vi "总磷氨氮插入数据.vi"(0 "table":string, 1 "关键参数":T1, 5 "data":T3={"时间标识"=timestamp(0 s since 1904-01-01), "测量模式"=enum."水样测试", "数据标记表"="N", "监测值"=0.0, "单位"=0, "数据标识"="", "因子编码"=0, "标样参考值"=0.0, "F0"=0.0, "F1"=0.0, "F2"=0.0, "F3"=0.0, "F4"=0.0, "F5"=0.0, "F6"=0.0, "F7"=0.0, "X"=0.0, "温度"=0.0, "湿度"=0.0, "量程标识"="", "SN"="", "跨度值"=0.0} {"单位" items=["μg/L", "mg/L", "ppm", "mg/m3", "cm", "ppb", "μg/m3", "%", "nmol/mol", "μmol/mol", "MPN/L", "MPN/100ml", "ng/m3", "NTU", "无量纲", "ms/cm", "μs/cm"]}, 11 "error in (no error)":errorcluster) -> (15 "error out":errorcluster)   [LabVIEW 2016, in "斯坦道氨氮.lvlib"]
uses:
  <vilib>/Utility/sysdir.llb/System Directory Type.ctl
  <vilib>/Utility/error.llb/DialogType.ctl
  <vilib>/addons/database/Auxilliary.llb/DB Tools Column Info.ctl
  <vilib>/addons/database/Auxilliary.llb/DB Tools DataTypes.ctl
  <vilib>/addons/database/Connection.llb/DB Tools Open Connec (String).vi
  <vilib>/addons/database/Connection.llb/Conn Execute.vi
  <vilib>/addons/database/Recordset.llb/Rec Fetch Recordset Data (R).vi
  <vilib>/addons/database/Recordset.llb/Rec Destroy - Connection.vi
  <vilib>/addons/database/NI_Database_API.lvlib
  <vilib>/Utility/VariantDataType/VariantType.lvlib
panel:
  out "data输出":T2
  out "为空？":bool
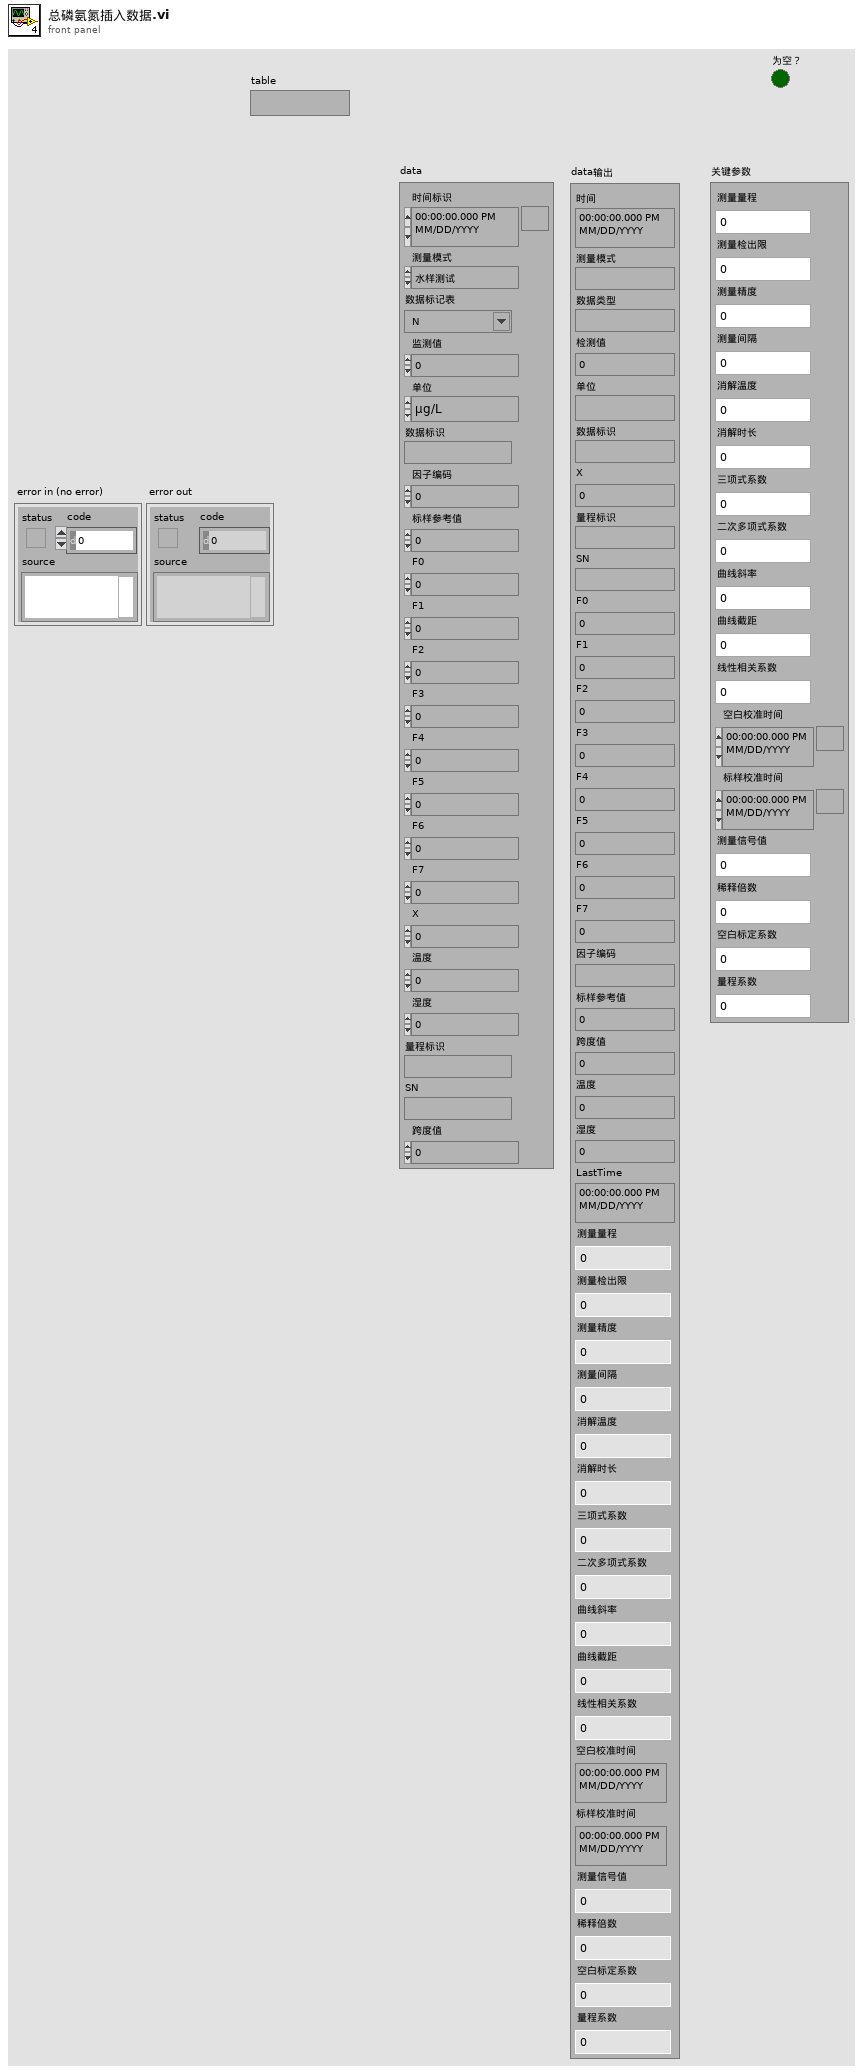
[diagram p1: front panel]
types:
  T1 = typedef "斯坦道氨氮.lvlib/关键参数.ctl" = cluster{"测量量程":sgl, "测量检出限":sgl, "测量精度":sgl, "测量间隔":sgl, "消解温度":sgl, "消解时长":sgl, "三项式系数":sgl, "二次多项式系数":sgl, "曲线斜率":sgl, "曲线截距":sgl, "线性相关系数":sgl, "空白校准时间":timestamp, "标样校准时间":timestamp, "测量信号值":sgl, "稀释倍数":sgl, "空白标定系数":sgl, "量程系数":sgl}
  T2 = cluster{"时间":timestamp, "测量模式":string, "数据类型":string, "检测值":sgl, "单位":string, "数据标识":string, "X":sgl, "量程标识":string, "SN":string, "F0":sgl, "F1":sgl, "F2":sgl, "F3":sgl, "F4":sgl, "F5":sgl, "F6":sgl, "F7":sgl, "因子编码":string, "标样参考值":sgl, "跨度值":sgl, "温度":sgl, "湿度":sgl, "LastTime":timestamp, "测量量程":sgl, "测量检出限":sgl, "测量精度":sgl, "测量间隔":sgl, "消解温度":sgl, "消解时长":sgl, "三项式系数":sgl, "二次多项式系数":sgl, "曲线斜率":sgl, "曲线截距":sgl, "线性相关系数":sgl, "空白校准时间":timestamp, "标样校准时间":timestamp, "测量信号值":sgl, "稀释倍数":sgl, "空白标定系数":sgl, "量程系数":sgl}
  T3 = cluster{"时间标识":timestamp, "测量模式":enum16{"维护数据", "水样测试", "标样核查", "零点核查", "跨度核查", "空白测试", "平行样测试", "加标回收", "空白校准", "标样校准", "初始化（清洗）", "快捷测试"}, "数据标记表":string, "监测值":sgl, "单位":u16, "数据标识":string, "因子编码":u32, "标样参考值":sgl, "F0":sgl, "F1":sgl, "F2":sgl, "F3":sgl, "F4":sgl, "F5":sgl, "F6":sgl, "F7":sgl, "X":sgl, "温度":sgl, "湿度":sgl, "量程标识":string, "SN":string, "跨度值":sgl}
  T4 = typedef "DialogType.ctl" = u16
  T5 = typedef "System Directory Type.ctl" = i32
  T6 = typedef "NI_Database_API.lvlib/Conn ObjectReference.ctl" = refnum<k1>
  T7 = typedef "NI_Database_API.lvlib/Rec ObjectReference.ctl" = refnum<k1>
  T8 = cluster{"测量量程":dbl, "测量精度":dbl, "测量间隔":dbl, "消解温度":dbl, "消解时长":dbl, "空白校准时间":timestamp, "曲线截距":dbl, "曲线斜率":dbl, "测量检出限":dbl, "测量信号值":dbl, "线性相关系数":dbl, "二次多项式系数":dbl, "标样校准时间":timestamp, "稀释倍数":dbl, "三项式系数":dbl, "空白标定系数":dbl, "量程系数":dbl, "F0/ORPA":dbl, "F1/ORPB":dbl, "F2/ORPK":dbl, "F3":dbl, "F4":dbl, "F5":dbl, "F6":dbl, "F7":dbl, "X0/滴定数":dbl, "量程":dbl}
  T9 = typedef "NI_Database_API.lvlib/DB Tools Column Info.ctl" = cluster{"column name":string, "data type":T10, "size":i32, "allow null?":bool}
  T10 = typedef "NI_Database_API.lvlib/DB Tools DataTypes.ctl" = enum16{"String", "Long (I32)", "Single (SGL)", "Double (DBL)", "Date/Time", "Binary"}
  T11 = typedef "VariantType.lvlib/Type.ctl" = enum8{"Invalid Type", "Void", "I8", "I16", "I32", "I64", "U8", "U16", "U32", "U64", "Single Float", "Double Float", "Extended Float", "Single Complex", "Double Complex", "Extended Complex", "Enum U8", "Enum U16", "Enum U32", "Enum U64", "Single Float With Unit", "Double Float With Unit", "Extended Float With Unit", "Single Complex with Unit", "Double Complex with Unit", "Extended Complex with Unit", "Boolean", "String", "Path", "Picture", "Tag", "Array", "Cluster", "Variant", "LV Variant", "Waveform", "Timestamp", "Digital Waveform", "Digital Data", "ExpressData", "Refnum", "External Data", "VI", "Poly VI", "LabVIEW Class Instance", "Fixed Point"}
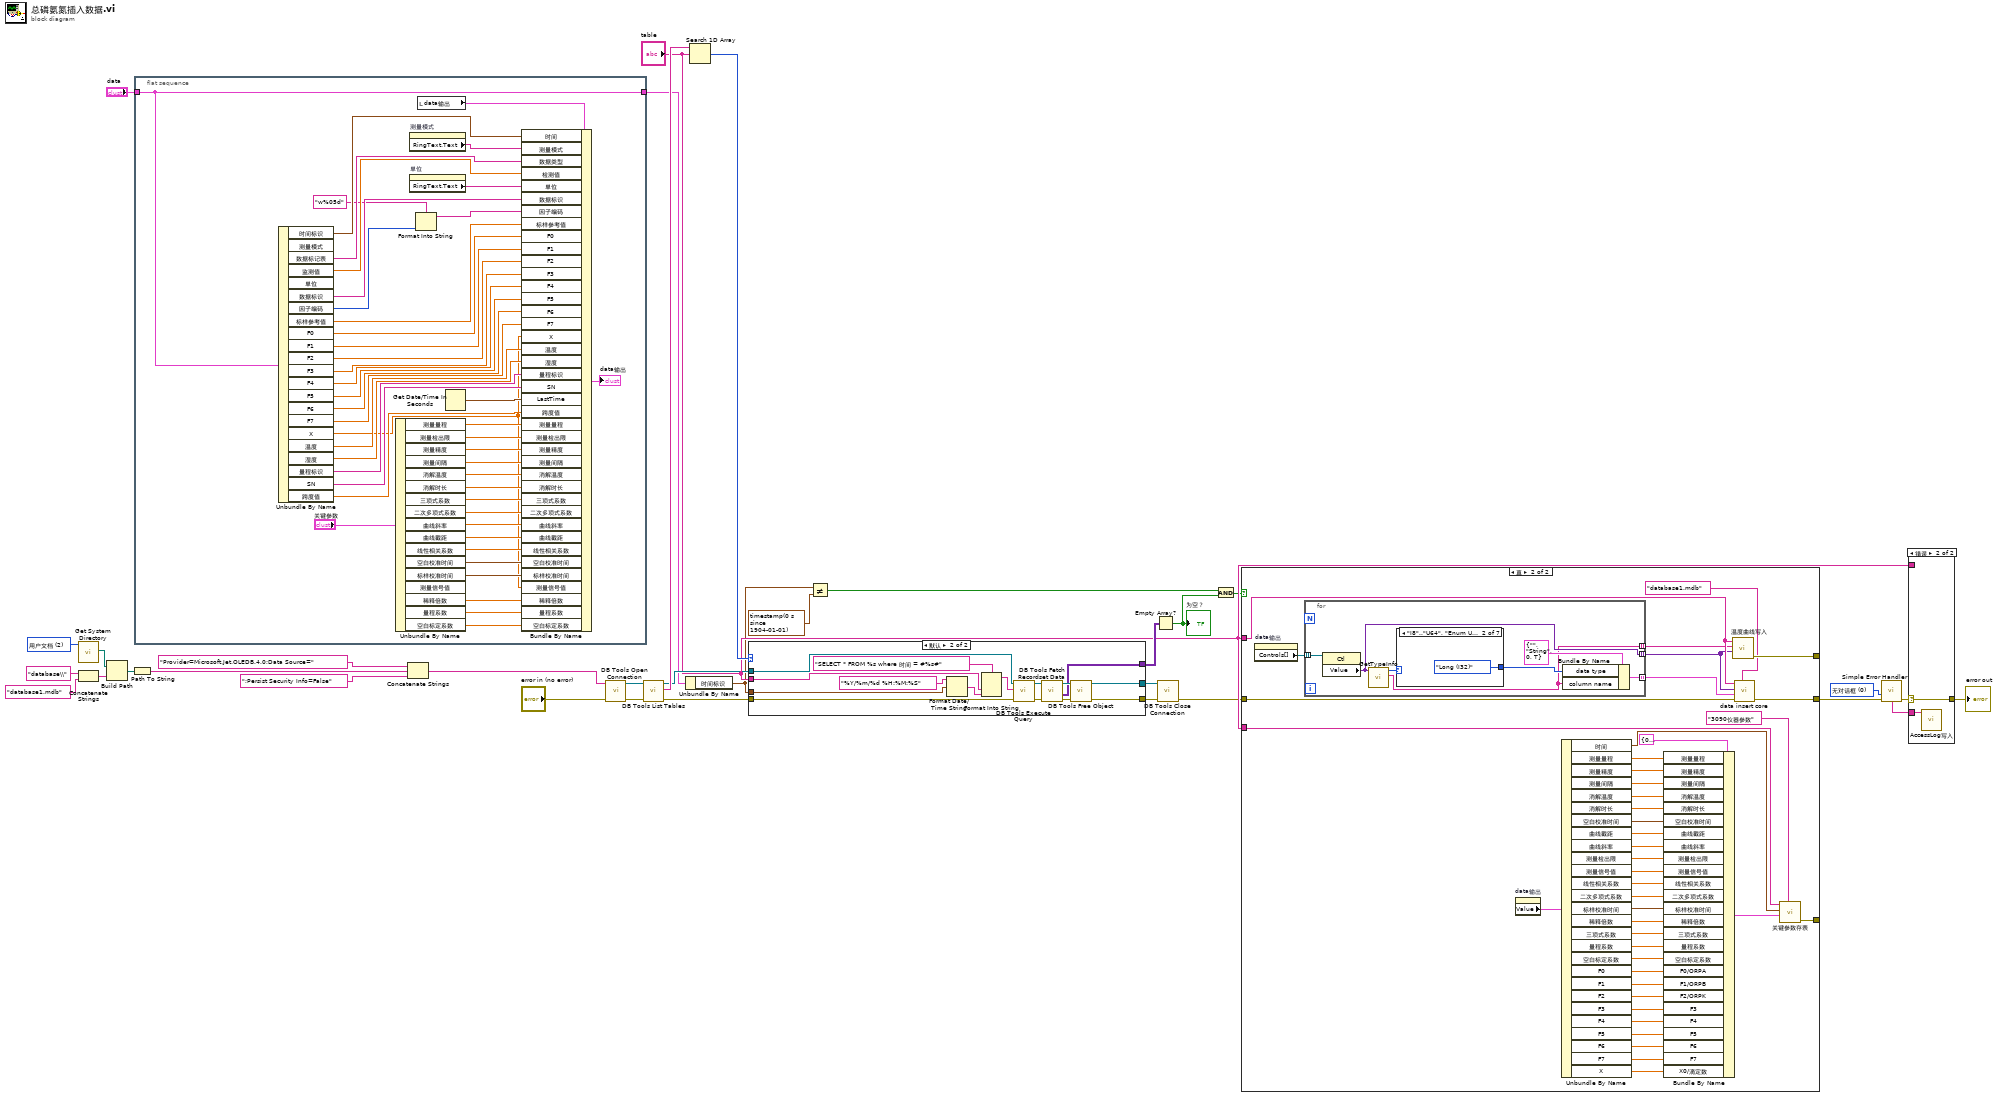
[diagram p0: block diagram]
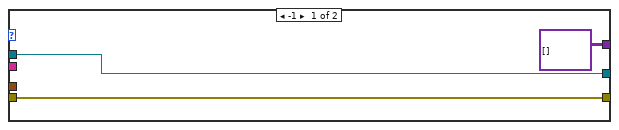
[diagram p3: hidden frame]
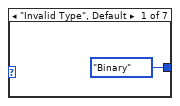
[diagram p5: hidden frame]
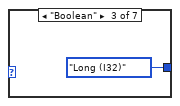
[diagram p6: hidden frame]
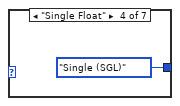
[diagram p7: hidden frame]
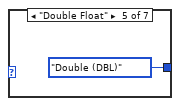
[diagram p8: hidden frame]
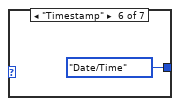
[diagram p9: hidden frame]
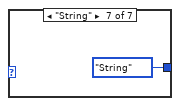
[diagram p10: hidden frame]
diagram:
  w15 = T4 0 items=["无对话框", "确定信息", "继续或停止信息", "确定信息＋警告", "继续/停止+警告"] ("type of dialog (OK msg:1)")
  w33 = T5 2 items=["用户目录"=0, "用户桌面"=1, "用户文档"=2, "用户应用程序数据"=3, "用户设置"=4, "用户临时目录"=5, "公共文档"=6, "公共应用程序数据"=7, "公共设置"=8, "公共缓存"=13, "系统核心库"=9, "系统安装库"=10, "应用程序文件"=11, "启动盘根目录"=12] ("system directory type")
  n1 = call <vilib>:"Get System Directory.vi"("system directory type"=w33) -> ("system directory"=w31:path)  [unwired: 10 in]
  n2 = Concatenate Strings("database\\" ("condition"), "database1.mdb" ("database")) -> (w25:string)
  n3 = Build Path(base path=w31, name or relative path=w25) -> (appended path=w30:path)
  n4 = Path To String(path=w30) -> (string=w29:string)
  n5 = flat-sequence {
    tunnel: "data" -> [w58]
    tunnel: [w58] -> w9
    frame #0 {
      n6 = Unbundle By Name(w58) -> ("时间标识"=w78:timestamp, "数据标记表"=w76:string, "监测值"=w75:sgl, "数据标识"=w73:string, "因子编码"=w57:u32, "标样参考值"=w72:sgl, "F0"=w71:sgl, "F1"=w70:sgl, "F2"=w69:sgl, "F3"=w68:sgl, "F4"=w67:sgl, "F5"=w66:sgl, "F6"=w65:sgl, "F7"=w64:sgl, "X"=w36:sgl, "温度"=w63:sgl, "湿度"=w62:sgl, "量程标识"=w61:string, "SN"=w60:string, "跨度值"=w53:sgl)  [unwired: 2 out]
      n7 = Unbundle By Name("关键参数") -> ("测量量程"=w51:sgl, "测量检出限"=w50:sgl, "测量精度"=w49:sgl, "测量间隔"=w48:sgl, "消解温度"=w47:sgl, "消解时长"=w46:sgl, "三项式系数"=w45:sgl, "二次多项式系数"=w44:sgl, "曲线斜率"=w43:sgl, "曲线截距"=w42:sgl, "线性相关系数"=w41:sgl, "空白校准时间"=w40:timestamp, "标样校准时间"=w39:timestamp, "稀释倍数"=w38:sgl, "量程系数"=w37:sgl, "空白标定系数"=w35:sgl)  [unwired: 1 out]
      n8 = property on="测量模式" class="Enum (严格)"() -> ("RingText.Text"=w77:string)  [unwired: 2 in, 2 out]
      n9 = property on="单位" class="Ring (严格)"() -> ("RingText.Text"=w74:string)  [unwired: 2 in, 2 out]
      n10 = Format Into String(format string="w%05d" ("格式字符串"), w57) -> (resulting string=w55:string)  [unwired: 2 in, 1 out]
      n11 = local read "data输出"() -> (w54:T2)
      n12 = Get Date/Time In Seconds() -> (seconds since 1Jan1904=w59:timestamp)
      n13 = Bundle By Name(cluster=w54, "时间"=w78, "测量模式"=w77, "数据类型"=w76, "检测值"=w75, "单位"=w74, "数据标识"=w73, "因子编码"=w55, "标样参考值"=w72, "F0"=w71, "F1"=w70, "F2"=w69, "F3"=w68, "F4"=w67, "F5"=w66, "F6"=w65, "F7"=w64, "X"=w36, "温度"=w63, "湿度"=w62, "量程标识"=w61, "SN"=w60, "LastTime"=w59, "跨度值"=w53, "测量量程"=w51, "测量检出限"=w50, "测量精度"=w49, "测量间隔"=w48, "消解温度"=w47, "消解时长"=w46, "三项式系数"=w45, "二次多项式系数"=w44, "曲线斜率"=w43, "曲线截距"=w42, "线性相关系数"=w41, "空白校准时间"=w40, "标样校准时间"=w39, "测量信号值"=w36, "稀释倍数"=w38, "量程系数"=w37, "空白标定系数"=w35) -> (→"data输出":T2)
    }
  }
  n14 = Concatenate Strings("Provider=Microsoft.Jet.OLEDB.4.0;Data Source=" ("condition"), w29, ";Persist Security Info=False" ("condition")) -> (w27:string)
  n15 = call-poly <vilib>:"DB Tools Open Connection.vi"("error in (no error)"="error in (no error)", "connection information"=w27) -> ("error out"=w23:errorcluster, "connection reference"=w24:T6)  [unwired: 6 in]
  n16 = call <vilib>:"DB Tools List Tables.vi"("error in (no error)"=w23, "connection reference"=w24) -> ("error out"=w17:errorcluster, "tables"=w22:string[], "connection reference out"=w18:T6)  [unwired: 3 in]
  n17 = Unbundle By Name(w9) -> ("时间标识"=w7:timestamp)
  n18 = Search 1D Array(1D array=w22, element="table") -> (index of element=w19:i32)  [unwired: 1 in]
  n19 = case shown="默认" w19 {
    tunnel: [variant[][] [] ("recordset data") w93] -> w16
    tunnel: [w82 w84] -> w4
    tunnel: [w81 w92] -> w3
    tunnel: w18 -> [w82 w88]
    tunnel: w17 -> [w81 w87]
    tunnel: "table" -> [_ w86]
    tunnel: w7 -> [_ w83]
    frame -1 {
    }
    frame Default {
      n20 = Format Date/Time String(time format string (%c)="%Y/%m/%d %H:%M:%S" ("时间格式字符串(%c)"), seconds (now)=w83) -> (date/time string=w89:string)  [unwired: 1 in]
      n21 = Format Into String(format string="SELECT * FROM %s where 时间 = #%s#" ("格式字符串"), w86, w89) -> (resulting string=w91:string)  [unwired: 2 in, 1 out]
      n22 = call-poly <vilib>:"DB Tools Execute Query.vi"("error in (no error)"=w87, "SQL query"=w91, "connection reference"=w88) -> ("error out"=w94:errorcluster, "recordset reference"=w97:T7)  [unwired: 5 in]
      n23 = call-poly <vilib>:"DB Tools Fetch Recordset Data.vi"("error in (no error)"=w94, "recordset reference"=w97) -> ("error out"=w95:errorcluster, "recordset data"=w93:variant[][], "recordset reference out"=w96:T7)  [unwired: 3 in]
      n24 = call-poly <vilib>:"DB Tools Free Object.vi"("error in (no error)"=w95, "recordset reference"=w96) -> ("error out"=w92:errorcluster, "connection reference"=w84:T6)  [unwired: 8 in]
    }
  }
  n25 = Not Equal?(x=w7, y=timestamp(0 s since 1904-01-01)) -> (x != y?=w5:bool)
  n26 = Empty Array?(array=w16) -> (empty?=w20:bool)
  "为空？" <- w20
  n27 = call <vilib>:"DB Tools Close Connection.vi"("error in (no error)"=w3, "connection reference"=w4) -> ("error out"=w2:errorcluster)  [unwired: 5 in]
  n28 = And(x=w5, y=w20) -> (x .and. y?=w6:bool)
  n29 = case shown="真" w6 {
    tunnel: "table" -> [_ w135]
    tunnel: w2 -> [w98 w136]
    tunnel: [w98 w139] -> w1
    tunnel: "table" -> [_ w140]
    tunnel: [_ w134] -> _
    tunnel: [_ w127] -> _
    frame False {
    }
    frame True {
      n30 = property on="data输出" class="Clust (严格)"() -> ("Controls[]"=w138:refnum<vi>[])  [unwired: 2 in, 2 out]
      n31 = for {
        tunnel: w138 -> [w147] mode=indexing
        tunnel: [w142] -> w132 mode=indexing
        tunnel: [w143] -> w137 mode=indexing
        tunnel: [w141] -> w133 mode=indexing
        n32 = property class="Ctl"(reference=w147) -> ("Value"=w142:variant)  [unwired: 1 in, 2 out]
        n33 = call <vilib>:"GetTypeInfo.vi"("Variant"=w142) -> ("Name"=w141:string, "Type Enum"=w145:T11)  [unwired: 6 in, 3 out]
        n34 = case shown="\"I8\"..\"U64\", \"Enum U8\"..\"Enum U64\"" w145 {
          tunnel: [DB_Tools_DataTypes."Binary" ("data type") DB_Tools_DataTypes."Long (I32)" ("data type") DB_Tools_DataTypes."Long (I32)" ("data type") DB_Tools_DataTypes."Single (SGL)" ("data type") DB_Tools_DataTypes."Double (DBL)" ("data type") DB_Tools_DataTypes."Date/Time" ("data type") DB_Tools_DataTypes."String" ("data type")] -> w144
          frame "Invalid Type", Default {
          }
          frame "I8".."U64", "Enum U8".."Enum U64" {
          }
          frame "Boolean" {
          }
          frame "Single Float" {
          }
          frame "Double Float" {
          }
          frame "Timestamp" {
          }
          frame "String" {
          }
        }
        n35 = Bundle By Name(cluster=T9 {"column name"="", "data type"=enum."String", "size"=0, "allow null?"=TRUE} ("column information"), "data type"=w144, "column name"=w141) -> (w143:T9)
      }
      n36 = property on="data输出" class="Clust (严格)"() -> ("Value"=w126:T2)  [unwired: 2 in, 2 out]
      n37 = Unbundle By Name(w126) -> ("时间"=w125:timestamp, "测量量程"=w99:sgl, "测量精度"=w100:sgl, "测量间隔"=w101:sgl, "消解温度"=w102:sgl, "消解时长"=w103:sgl, "空白校准时间"=w104:timestamp, "曲线截距"=w105:sgl, "曲线斜率"=w106:sgl, "测量检出限"=w107:sgl, "测量信号值"=w108:sgl, "线性相关系数"=w109:sgl, "二次多项式系数"=w110:sgl, "标样校准时间"=w111:timestamp, "稀释倍数"=w112:sgl, "三项式系数"=w113:sgl, "量程系数"=w114:sgl, "空白标定系数"=w115:sgl, "F0"=w116:sgl, "F1"=w117:sgl, "F2"=w118:sgl, "F3"=w119:sgl, "F4"=w120:sgl, "F5"=w121:sgl, "F6"=w122:sgl, "F7"=w123:sgl, "X"=w124:sgl)
      n38 = Bundle By Name(cluster=T8 {"测量量程"=0.0, "测量精度"=0.0, "测量间隔"=0.0, "消解温度"=0.0, "消解时长"=0.0, "空白校准时间"=timestamp(0 s since 1904-01-01), "曲线截距"=0.0, "曲线斜率"=0.0, "测量检出限"=0.0, "测量信号值"=0.0, "线性相关系数"=0.0, "二次多项式系数"=0.0, "标样校准时间"=timestamp(0 s since 1904-01-01), "稀释倍数"=0.0, "三项式系数"=0.0, "空白标定系数"=0.0, "量程系数"=0.0, "F0/ORPA"=0.0, "F1/ORPB"=0.0, "F2/ORPK"=0.0, "F3"=0.0, "F4"=0.0, "F5"=0.0, "F6"=0.0, "F7"=0.0, "X0/滴定数"=0.0, "量程"=0.0} ("仪器参数"), "测量量程"=w99, "测量精度"=w100, "测量间隔"=w101, "消解温度"=w102, "消解时长"=w103, "空白校准时间"=w104, "曲线截距"=w105, "曲线斜率"=w106, "测量检出限"=w107, "测量信号值"=w108, "线性相关系数"=w109, "二次多项式系数"=w110, "标样校准时间"=w111, "稀释倍数"=w112, "三项式系数"=w113, "量程系数"=w114, "空白标定系数"=w115, "F0/ORPA"=w116, "F1/ORPB"=w117, "F2/ORPK"=w118, "F3"=w119, "F4"=w120, "F5"=w121, "F6"=w122, "F7"=w123, "X0/滴定数"=w124) -> (w128:T8)
      n39 = call "温度曲线写入.vi"("属性值"=w132, "属性名称"=w133, "table"=w135) -> ("错误输出"=w134:errorcluster)  [unwired: 8 in]
      n40 = call "data insert core.vi"("database"="database1.mdb", "error in (no error)"=w136, "column information"=w137, "data"=w132, "table"=w135) -> ("error out"=w139:errorcluster)  [unwired: 6 in]
      n41 = call "关键参数存表.vi"("table"="3090仪器参数", "仪器参数"=w128, "datatime"=w125, "仪器名称"=w140) -> ("error out"=w127:errorcluster)  [unwired: 7 in]
    }
  }
  n42 = call <vilib>:"Simple Error Handler.vi"("type of dialog (OK msg:1)"=w15, "error in (no error)"=w1) -> ("error out"=w14:errorcluster, "message"=w13:string)  [unwired: 3 in, 3 out]
  n43 = case shown="错误" w14 {
    selector: w14 -> [_ w155]
    tunnel: w13 -> [_ w156]
    tunnel: [_ w155] -> w12
    tunnel: "table" -> [_ _]
    frame No Error {
    }
    frame Error {
      n44 = call "AccessLog写入.vi"("Log"=w156) -> ()  [unwired: 11 in]
    }
  }
  "error out" <- w12
